vi "Initialize.vi"(8 "error in (no error)":errorcluster, 11 "initialization in":refnum<class "initializable.lvclass">) -> (0 "error out":errorcluster, 3 "initialization out":refnum<class "initializable.lvclass">)   [LabVIEW 2020, in "eos.lvlib" / "initializable.lvclass"]
uses:
  initializable.lvclass
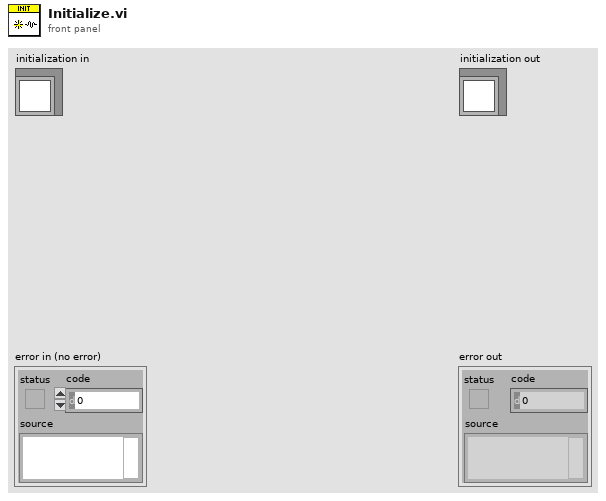
[diagram p1: front panel]
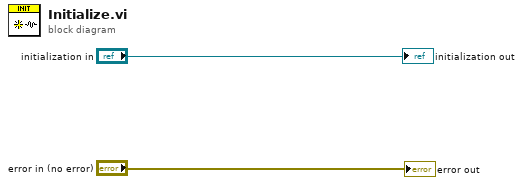
[diagram p0: block diagram]
diagram:
  "error out" <- "error in (no error)"
  "initialization out" <- "initialization in"
